vi "CSM Application Directory.vi"() -> (2 "CSM Application Dir":path)   [LabVIEW 2017, in "CSM File Logger.lvlib"]
uses:
  CSM File Logger.lvlib
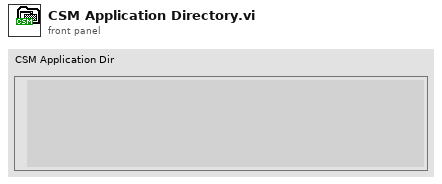
[diagram p1: front panel]
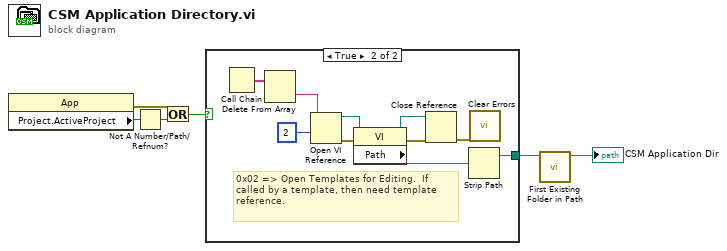
[diagram p0: block diagram]
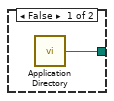
[diagram p2: hidden frame]
diagram:
  n1 = property class="App"() -> (error out=w6:errorcluster, "Project.ActiveProject"=w4:refnum<vi>)  [unwired: 2 in, 1 out]
  n2 = Not A Number/Path/Refnum?(number/path/refnum=w4) -> (NaN/Path/Refnum?=w5:bool)
  n3 = Or(x=w6, y=w5) -> (x .or. y?=w3:bool)
  n4 = case shown="True" w3 {
    tunnel: [w7 w8] -> w2
    frame False {
      n5 = call <vilib>:"Application Directory.vi"() -> ("Application Directory"=w7:path)
    }
    frame True {
      # "0x02 => Open Templates for Editing.  If called by a template, then need template reference."
      n6 = Call Chain() -> (call chain=w13:string[])
      n7 = Delete From Array(array=w13) -> (deleted portion=w12:string)  [unwired: 2 in, 1 out]
      n8 = Open VI Reference(vi path=w12, options=2) -> (vi reference=w10:refnum<vi>, error out=w14:errorcluster)  [unwired: 4 in]
      n9 = property class="VI"(reference=w10, error in=w14) -> (reference out=w16:refnum<vi>, error out=w15:errorcluster, "Path"=w9:path)
      n10 = Close Reference(reference=w16, error in (no error)=w15) -> (error out=w17:errorcluster)
      n11 = Strip Path(path=w9) -> (stripped path=w8:path)  [unwired: 1 out]
      n12 = call <vilib>:"Clear Errors.vi"("error in (no error)"=w17) -> ()  [unwired: 5 in, 2 out]
    }
  }
  n13 = call "First Existing Folder in Path.vi"("Stripped Path In"=w2) -> ("Stripped Path Out"=→"CSM Application Dir":path)  [unwired: 10 in]
